vi "main.vi"() -> ()   [LabVIEW 2014]
uses:
  <vilib>/MakerHub/LINX/Public/Peripherals/Analog/Analog Read 1 Chan.vi
  <vilib>/MakerHub/LINX/Public/Peripherals/Analog/Analog Read N Chans.vi
  <vilib>/MakerHub/LINX/Private/Local IO/LinxAnalogRead.vi
  <vilib>/MakerHub/LINX/Public/Utilities/Check Channel.vi
  <vilib>/MakerHub/LINX/Private/Local IO/Handle Errors.vi
  <vilib>/MakerHub/LINX/Public/Utilities/Open Local.vi
  <vilib>/MakerHub/LINX/Private/Utilties/Generate Error.vi
  Global.vi
  <vilib>/MakerHub/LINX/LMH-LINX.lvlib
panel:
  out "Voltage":dbl
  out "State":T1(ring)
  out "Error Out":errorcluster
  in  "stop":bool
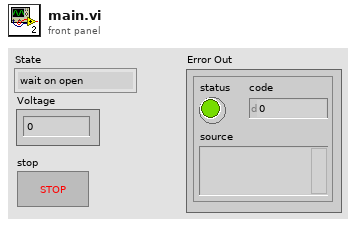
[diagram p1: front panel]
types:
  T1 = enum16{"wait on open", "debounce open", "wait on close", "debounce close", "decrement counter"}
  T2 = typedef "LMH-LINX.lvlib/LINX Ref.ctl" = cluster{"IO":T3, "Interface":T4, "LINX Device Config":T5}
  T3 = typedef "LMH-LINX.lvlib/Platform.ctl" = enum16{"Remote", "Local"}
  T4 = typedef "LMH-LINX.lvlib/Interface.ctl" = enum16{"Serial", "TCP"}
  T5 = typedef "LMH-LINX.lvlib/Device.lvlib/LINX Device Config.ctl" = cluster{"Interface":T4, "COM Port":refnum<visa-resource-name>, "TCP Configuration":T6, "Device Family":u8, "Device ID":u8, "Device Name":string, "TCP Ref":refnum<k5>, "Channels":T7}
  T6 = typedef "LMH-LINX.lvlib/Device.lvlib/TCP Config.ctl" = cluster{"IP Address":string, "Port":u16}
  T7 = typedef "LMH-LINX.lvlib/Channels.ctl" = cluster{"DI":u8[], "DO":u8[], "AI":u8[], "AO":u8[], "PWM":u8[], "QE":u8[], "UART":u8[], "I2C 2":u8[], "SPI":u8[], "CAN":u8[], "Servo":u8[], "AI Ref (V)":dbl, "AI Resolution (Bits)":u8, "AO Ref (V)":dbl, "AO Resolution (Bits)":u8}
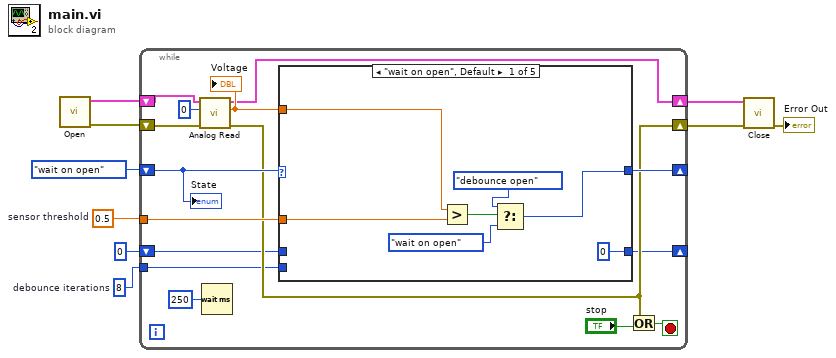
[diagram p0: block diagram]
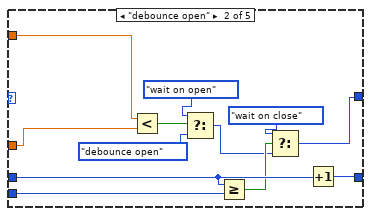
[diagram p2: hidden frame]
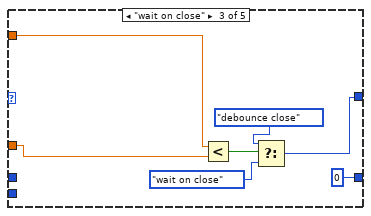
[diagram p3: hidden frame]
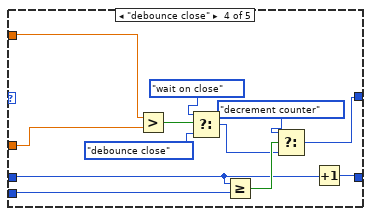
[diagram p4: hidden frame]
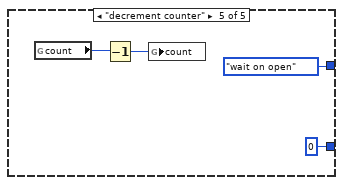
[diagram p5: hidden frame]
diagram:
  w1 = 8  # debounce iterations
  w3 = 0.5  # sensor threshold
  n1 = call-poly <vilib>:"Open.vi"() -> ("Error Out"=w7:errorcluster, "LINX Resource"=w8:T2)  [unwired: 9 in, 1 out]
  n2 = while {
    shift-right: [w13] -> w6
    shift-left: w7 -> [w15]
    shift-right: [w19] -> _
    shift-left: T1."wait on open" -> [w24]
    tunnel: w3 -> [w21]
    shift-right: [w14] -> w5
    shift-left: w8 -> [w16]
    shift-right: [w11] -> _
    shift-left: 0 -> [w12]
    tunnel: w1 -> [w10]
    stop <- w22 stop-if-true
    n3 = call-poly <vilib>:"Analog Read.vi"("Error In"=w15, "Analog Channel"=u8 0, "LINX Resource"=w16) -> ("Error Out"=w13:errorcluster, "Voltage"=w17:dbl, "LINX Resource"=w14:T2)  [unwired: 5 in, 1 out]
    "Voltage" <- w17
    n4 = Wait (ms)(milliseconds to wait=u32 250) -> ()  [unwired: 1 out]
    n5 = case shown="\"wait on open\", Default" w24 {
      tunnel: w21 -> [w31 w38 w45 w54 _]
      tunnel: [w27 w32 w44 w51 T1."wait on open"] -> w19
      tunnel: w17 -> [w26 w39 w46 w53 _]
      tunnel: w12 -> [_ w36 _ w56 _]
      tunnel: [0 w43 0 w52 0] -> w11
      tunnel: w10 -> [_ w37 _ w55 _]
      frame "wait on open", Default {
        n6 = Greater?(x=w26, y=w31) -> (0:w30:bool)
        n7 = Select(t=T1."debounce open", s=w30, f=T1."wait on open") -> (s? t:f=w27:T1)
      }
      frame "debounce open" {
        n8 = Less?(x=w39, y=w38) -> (x < y?=w42:bool)
        n9 = Select(t=T1."wait on open", s=w42, f=T1."debounce open") -> (s? t:f=w33:T1)
        n10 = Greater Or Equal?(x=w36, y=w37) -> (x >= y?=w35:bool)
        n11 = Select(t=T1."wait on close", s=w35, f=w33) -> (s? t:f=w32:T1)
        n12 = Increment(x=w36) -> (x+1=w43:i32)
      }
      frame "wait on close" {
        n13 = Less?(x=w46, y=w45) -> (x < y?=w50:bool)
        n14 = Select(t=T1."debounce close", s=w50, f=T1."wait on close") -> (s? t:f=w44:T1)
      }
      frame "debounce close" {
        n15 = Greater?(x=w53, y=w54) -> (0:w62:bool)
        n16 = Select(t=T1."wait on close", s=w62, f=T1."debounce close") -> (s? t:f=w57:T1)
        n17 = Greater Or Equal?(x=w56, y=w55) -> (x >= y?=w59:bool)
        n18 = Select(t=T1."decrement counter", s=w59, f=w57) -> (s? t:f=w51:T1)
        n19 = Increment(x=w56) -> (x+1=w52:i32)
      }
      frame "decrement counter" {
        n20 = global read "Global.vi" "count"() -> (w66:i32)
        n21 = Decrement(x=w66) -> (x-1=w65:i32)
        n22 = global write "Global.vi" "count"(w65) -> ()
      }
    }
    n23 = Or(x=w13, y="stop") -> (x .or. y?=w22:bool)
    "State" <- w24
  }
  n24 = call <vilib>:"Close.vi"("Error In"=w6, "LINX Resource"=w5) -> ("Error Out"=→"Error Out":errorcluster)  [unwired: 9 in]
